vi "写入DBL_B.vi"(8 "error in (no error)":errorcluster caption="错误输入（无错误）", 10 "DBL_B":dbl, 11 "运算类输入":refnum<class "运算类.lvclass">) -> (0 "error out":errorcluster caption="错误输出", 3 "运算类输出":refnum<class "运算类.lvclass">)   [LabVIEW 2013, in "运算类.lvclass"]
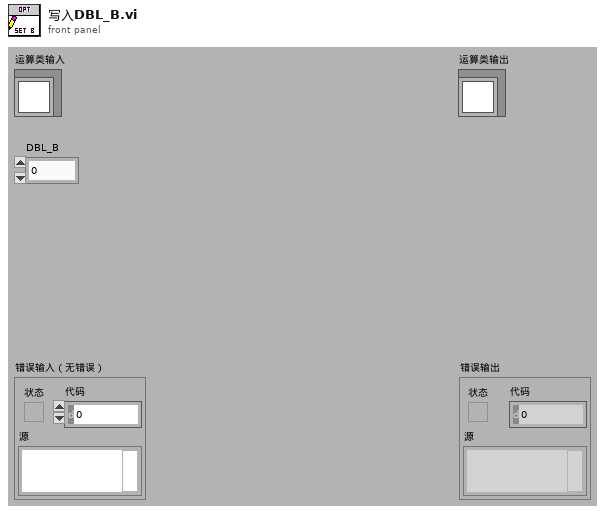
[diagram p1: front panel]
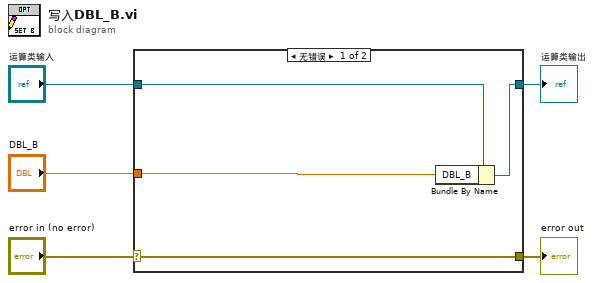
[diagram p0: block diagram]
diagram:
  n1 = case shown="无错误" "error in (no error)" {
    selector: "error in (no error)" -> [w9 w10]
    tunnel: [w9 w10] -> w4
    tunnel: [w7 w11] -> w2
    tunnel: "运算类输入" -> [w8 w11]
    tunnel: "DBL_B" -> [w6 _]
    frame No Error {
      n2 = Bundle By Name(cluster=w8, "DBL_B"=w6) -> (w7:refnum<class "运算类.lvclass">)
    }
    frame Error {
    }
  }
  "error out" <- w4
  "运算类输出" <- w2
